vi "Build Tree.vi"(8 "error in (no error)":errorcluster, 9 "Actual Path":path[](array[path]), 10 "Expected Path":path[](array[path]), 11 "Tree Refnum":refnum<vi>) -> (0 "error out":errorcluster, 3 "Tree Refnum out":refnum<vi>)   [LabVIEW 2023]
doc: "Populates the tree control identified by <B>Tree Refnum</B> with the other inputs, highlighting each row appropriately."
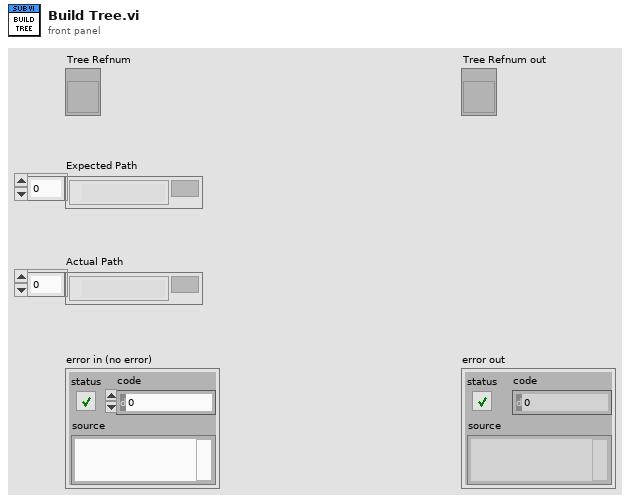
[diagram p1: front panel]
types:
  T1 = typedef "Tree Map Value.ctl" = cluster{"Tag":string, "Child Position":i32, "Actual Path":path}
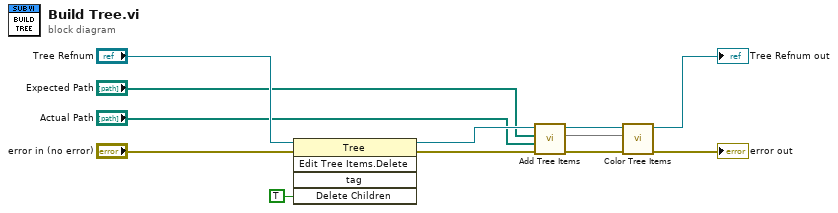
[diagram p0: block diagram]
diagram:
  n1 = invoke class="Tree" method="Edit Tree Items.Delete"(reference="Tree Refnum", error in="error in (no error)", "Delete Children"=TRUE ("Delete Children?")) -> (reference out=w9:refnum<vi>, error out=w8:errorcluster)  [unwired: 2 in, 3 out]
  n2 = call "Add Tree Items.vi"("error in (no error)"=w8, "Actual Path"="Actual Path", "Expected Path"="Expected Path", "Tree Refnum"=w9) -> ("error out"=w4:errorcluster, "Tree Map"=w5:map{path, T1}, "Tree Refnum out"=w10:refnum<vi>)  [unwired: 5 in]
  n3 = call "Color Tree Items.vi"("error in (no error)"=w4, "Tree Map"=w5, "Tree Refnum"=w10) -> ("error out"=→"error out":errorcluster, "Tree Refnum out"=→"Tree Refnum out":refnum<vi>)  [unwired: 7 in]
